vi "Single_pulse_ext_TTL.vi"() -> ()   [LabVIEW 2018]
uses:
  <vilib>/DAQmx/write.llb/DAQmx Write (Digital Bool 1Line 1Point).vi
  <vilib>/DAQmx/create/channels.llb/DAQmx Create Channel (DO-Digital Output).vi
  <vilib>/DAQmx/miscellaneous.llb/DAQmx Fill In Error Info.vi
panel:
  out "error out":errorcluster
  in  "Delay time, s":dbl min=0.0 max=5.0 step=0.1
  in  "Test":bool
  in  "Stop":bool
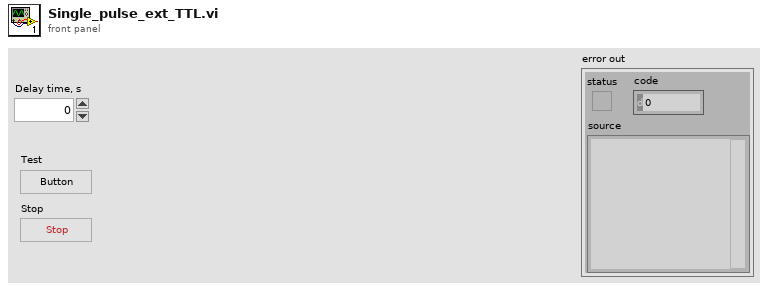
[diagram p1: front panel]
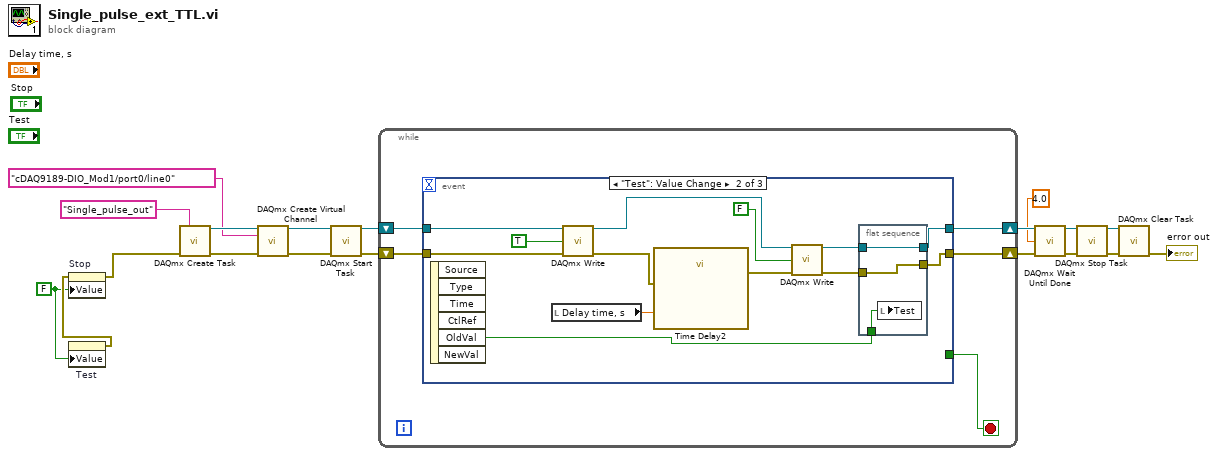
[diagram p0: block diagram]
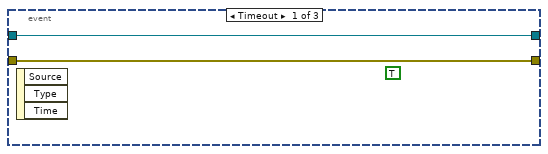
[diagram p2: hidden frame]
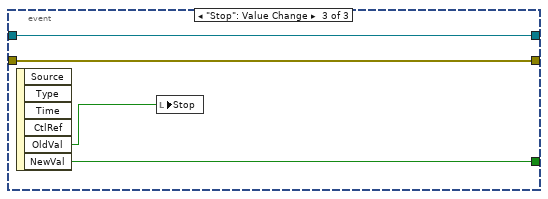
[diagram p3: hidden frame]
diagram:
  w2 = FALSE ("Stop")
  n1 = property on="Test" class="Bool (strict)"("Value"=w2) -> (error out=w3:errorcluster)  [unwired: 2 in, 1 out]
  n2 = property on="Stop" class="Bool (strict)"(error in=w3, "Value"=w2) -> (error out=w4:errorcluster)  [unwired: 1 in, 1 out]
  n3 = call <vilib>:"DAQmx Create Task.vi"("new task name"="Single_pulse_out", "error in"=w4) -> ("task out"=w18:refnum<k21>, "error out"=w17:errorcluster)  [unwired: 12 in]
  n4 = call-poly <vilib>:"DAQmx Create Virtual Channel.vi"("task in"=w18, "lines"=tag "cDAQ9189-DIO_Mod1/port0/line0", "error in"=w17) -> ("task out"=w13:refnum<k21>, "error out"=w15:errorcluster)  [unwired: 11 in]
  n5 = call <vilib>:"DAQmx Start Task.vi"("task/channels in"=w13, "error in"=w15) -> ("task out"=w12:refnum<k21>, "error out"=w14:errorcluster)  [unwired: 12 in]
  n6 = while {
    shift-right: [w21] -> w6
    shift-left: w14 -> [w24]
    shift-right: [w22] -> w7
    shift-left: w12 -> [w23]
    stop <- w20 stop-if-true
    n7 = event shown="[1] \"Test\": Value Change" {
      selector: _ -> [_ _ _]
      dyn-events: _ -> [_ _ _]
      timeout: _ -> [_ _ _]
      tunnel: w24 -> [w26 w34 w43]
      tunnel: w23 -> [w25 w33 w44]
      tunnel: [w25 w31 w44] -> w22
      tunnel: [w26 w29 w43] -> w21
      tunnel: [_ _ w45] -> w20
      event Timeout {
        (unwired) TRUE ("data")
        n8 = event-data() -> ()  [unwired: 1 in, 3 out]
      }
      event "Test": Value Change {
        n9 = event-data() -> ("OldVal"=w27:bool)  [unwired: 1 in, 5 out]
        n10 = local read "Delay time, s"() -> (w32:dbl)
        n11 = call-poly <vilib>:"DAQmx Write.vi"("task/channels in"=w33, "data"=TRUE, "error in"=w34) -> ("task out"=w36:refnum<k21>, "error out"=w38:errorcluster)  [unwired: 10 in, 1 out]
        n12 = call "Time Delay2"("error in (no error)"=w38, "Delay Time (s)"=w32) -> ("error out"=w37:errorcluster)  [unwired: 9 in]
        n13 = call-poly <vilib>:"DAQmx Write.vi"("task/channels in"=w36, "data"=FALSE, "error in"=w37) -> ("task out"=w30:refnum<k21>, "error out"=w28:errorcluster)  [unwired: 10 in, 1 out]
        n14 = flat-sequence {
          tunnel: [w42] -> w31
          tunnel: w30 -> [w42]
          tunnel: [w41] -> w29
          tunnel: w28 -> [w41]
          tunnel: w27 -> [w40]
          frame #0 {
            n15 = local write "Test"(w40) -> ()
          }
        }
      }
      event "Stop": Value Change {
        n16 = event-data() -> ("OldVal"=w46:bool, "NewVal"=w45:bool)  [unwired: 1 in, 4 out]
        n17 = local write "Stop"(w46) -> ()
      }
    }
  }
  n18 = call <vilib>:"DAQmx Wait Until Done.vi"("task/channels in"=w7, "timeout (sec)"=4.0, "error in"=w6) -> ("task out"=w9:refnum<k21>, "error out"=w8:errorcluster)  [unwired: 11 in]
  n19 = call <vilib>:"DAQmx Stop Task.vi"("task/channels in"=w9, "error in"=w8) -> ("task out"=w11:refnum<k21>, "error out"=w10:errorcluster)  [unwired: 12 in]
  n20 = call <vilib>:"DAQmx Clear Task.vi"("task in"=w11, "error in"=w10) -> ("error out"=→"error out":errorcluster)  [unwired: 13 in]
